vi "ExTestAdvDispOverlay.vi"() -> ()   [LabVIEW 2010]
panel:
  in  "Full File Name":path=path "C:/Program Files/SIToolKit/LabVIEW/Data Files/Ratso.TIF"
  out "error out":errorcluster
  in  "error in (no error)":errorcluster
  in  "SITKFULLDISPLAYLib.SITKFullDisplay":refnum<k7>(container)
  # "Use Ratso.tif for good example, it has two images to overlay"
  # "Browse match pattern is set to *.tif.  Modify this if different file type is needed."
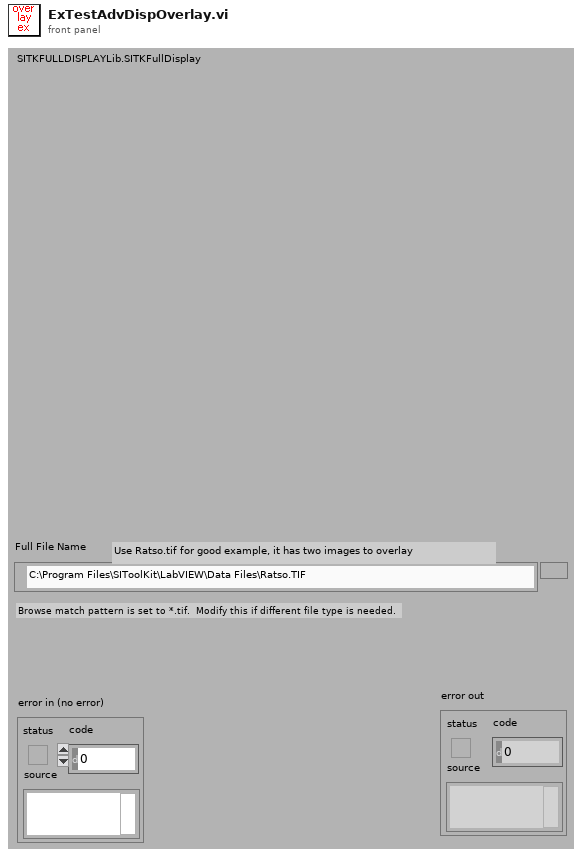
[diagram p1: front panel]
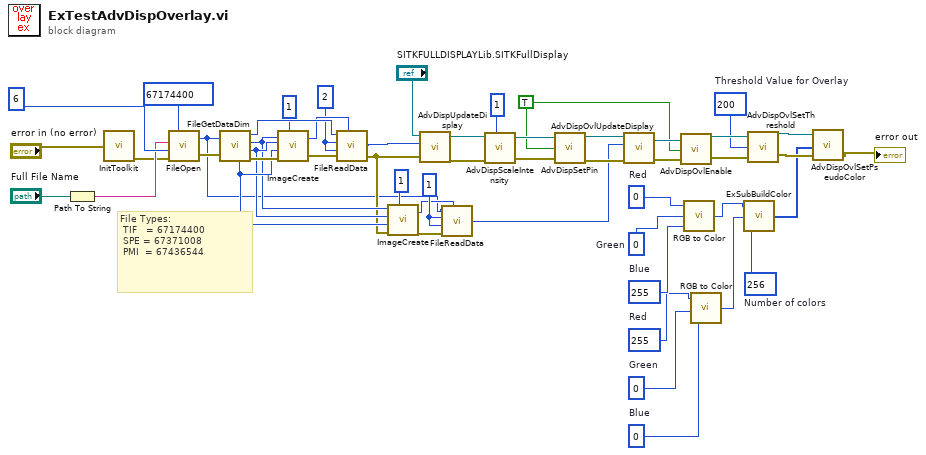
[diagram p0: block diagram]
diagram:
  w7 = 256  # Number of colors
  w11 = 0  # Blue
  w9 = 0  # Green
  w10 = 255  # Red
  w15 = 255  # Blue
  w14 = 0  # Green
  w13 = 0  # Red
  w16 = 200  # Threshold Value for Overlay
  w22 = 1
  w23 = 2
  w3 = TRUE
  # "File Types:\n TIF   = 67174400\n SPE = 67371008\n PMI  = 67436544"
  n1 = Path To String(path="Full File Name") -> (string=w48:string)
  n2 = call <userlib>:"InitToolkit.vi"("error in"="error in (no error)") -> ("error out"=w41:errorcluster)
  n3 = call <userlib>:"FileOpen.vi"("error in"=w41, "File Operations"=6, "FileName"=w48, "File Type"=67174400) -> ("error out"=w47:errorcluster, "File Handle"=w20:u32)
  n4 = call <userlib>:"FileGetDataDim.vi"("File Handle"=w20, "error in"=w47) -> ("Data Type"=w40:u32, "File Handle"=w45:u32, "X dim"=w38:u32, "Y dim"=w39:u32, "error out"=w46:errorcluster)  [unwired: 1 out]
  n5 = call <userlib>:"ImageCreate.vi"("X dimension"=w38, "Y dimension"=w39, "Data Type"=w40, "error in"=w46, "Number Of Frames"=1) -> ("Image Handle"=w43:u32, "error out"=w44:errorcluster)
  n6 = call <userlib>:"FileReadData.vi"("File Handle"=w45, "Start Frame"=w23, "End Frame"=w23, "error in"=w44, "Image Handle"=w43) -> ("Image Handle"=w27:u32, "error out"=w36:errorcluster)  [unwired: 1 out]
  n7 = call <userlib>:"ImageCreate.vi"("X dimension"=w38, "Y dimension"=w39, "Data Type"=w40, "error in"=w36, "Number Of Frames"=1) -> ("Image Handle"=w21:u32, "error out"=w25:errorcluster)
  n8 = call <userlib>:"AdvDispUpdateDisplay.vi"("error in (no error)"=w36, "Image Handle"=w27, "SITKFULLDISPLAYLib.SITKFullDisplay"="SITKFULLDISPLAYLib.SITKFullDisplay") -> ("error out"=w34:errorcluster, "SITKFULLDISPLAYLib.SITKFullDisplay"=w35:refnum<k7>)  [unwired: 1 in]
  n9 = call <userlib>:"FileReadData.vi"("File Handle"=w20, "Start Frame"=w22, "End Frame"=w22, "error in"=w25, "Image Handle"=w21) -> ("Image Handle"=w19:u32)  [unwired: 2 out]
  n10 = call <userlib>:"AdvDispScaleIntensity.vi"("SITKFULLDISPLAYLib.SITKFullDisplay"=w35, "error in (no error)"=w34, "Type of Scale"=1) -> ("SITKFULLDISPLAYLib.SITKFullDisplay"=w4:refnum<k7>, "error out"=w33:errorcluster)  [unwired: 2 in]
  n11 = call <userlib>:"AdvDispSetPin.vi"("SITKFULLDISPLAYLib.SITKFullDisplay"=w4, "Pin Enable"=w3, "error in (no error)"=w33) -> ("SITKFULLDISPLAYLib.SITKFullDisplay"=w29:refnum<k7>, "error out"=w31:errorcluster)  [unwired: 2 out]
  n12 = call <userlib>:"AdvDispOvlUpdateDisplay.vi"("error in (no error)"=w31, "Image Handle"=w19, "SITKFULLDISPLAYLib.SITKFullDisplay"=w29) -> ("error out"=w30:errorcluster, "SITKFULLDISPLAYLib.SITKFullDisplay"=w28:refnum<k7>)  [unwired: 1 in]
  n13 = call <userlib>:"AdvDispOvlEnable.vi"("error in (no error)"=w30, "Overlay Enable"=w3, "SITKFULLDISPLAYLib.SITKFullDisplay"=w28) -> ("error out"=w18:errorcluster, "SITKFULLDISPLAYLib.SITKFullDisplay"=w17:refnum<k7>)
  n14 = call <vilib>:"RGB to Color.vi"("B"=w15, "G"=w14, "R"=w13) -> ("Color"=w12:u32)
  n15 = call <vilib>:"RGB to Color.vi"("B"=w11, "G"=w9, "R"=w10) -> ("Color"=w8:u32)
  n16 = call "ExSubBuildColor.vi"("Count"=w7, "End Color"=w8, "Start Color"=w12) -> ("Array"=w5:i32[])
  n17 = call <userlib>:"AdvDispOvlSetThreshold.vi"("error in (no error)"=w18, "Threshold"=w16, "SITKFULLDISPLAYLib.SITKFullDisplay"=w17) -> ("error out"=w6:errorcluster, "SITKFULLDISPLAYLib.SITKFullDisplay"=w2:refnum<k7>)
  n18 = call <userlib>:"AdvDispOvlSetPseudoColor.vi"("error in (no error)"=w6, "Array"=w5, "SITKFULLDISPLAYLib.SITKFullDisplay"=w2) -> ("error out"=→"error out":errorcluster)  [unwired: 1 out]
